vi "测量文件.vi"() -> ()   [LabVIEW 2016]
panel:
  out "数值 8":dbl
  out "数值 7":dbl
  out "数值 6":dbl
  out "数值 5":dbl
  out "动态显示 2":dbl[](array[numeric])
  out "动态显示":dbl[](array[numeric])
  out "数值 4":dbl
  out "数值 3":dbl
  out "数值 2":dbl
  out "数值":dbl
  in  "conversion rate(Hz)":dbl
  in  "停止":bool
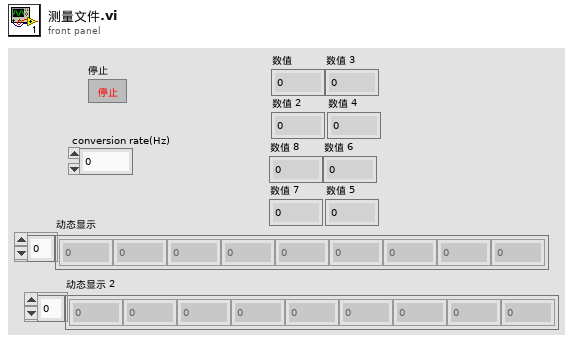
[diagram p1: front panel]
types:
  T1 = enum16{"open", "replace", "create", "open or create", "replace or create", "replace or create with confirmation"}
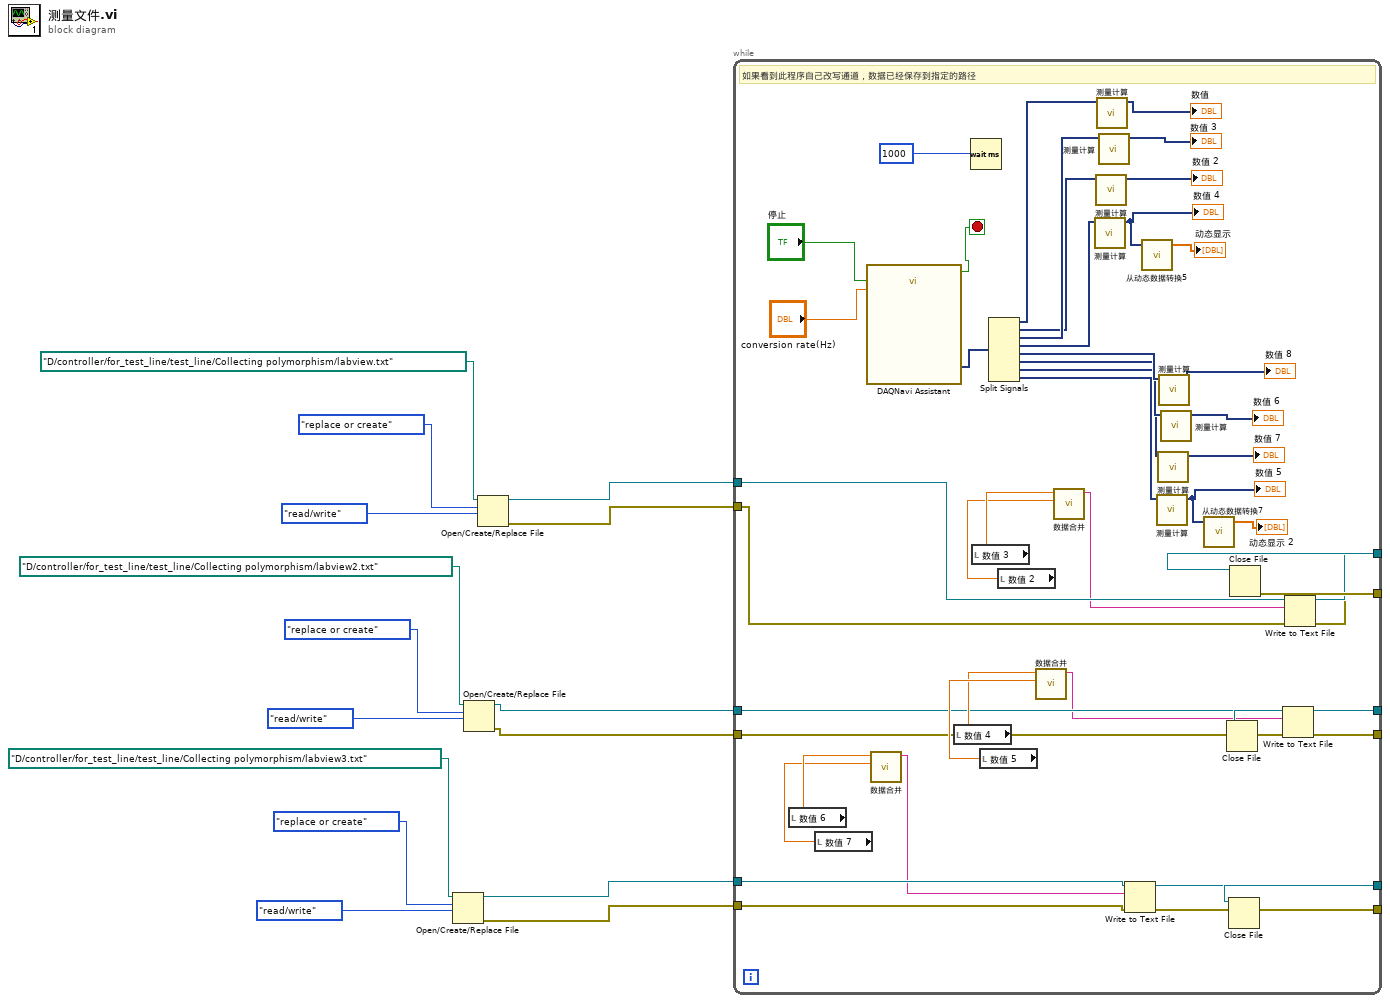
[diagram p0: block diagram]
diagram:
  n1 = Open/Create/Replace File(file path (use dialog)=path "D:/controller/for_test_line/test_line/Collecting polymorphism/labview3.txt" ("文件路径（使用对话框）"), operation (0:open)=T1."replace or create" ("操作(0:open)"), access (0:read/write)=enum16{"read/write", "read-only", "write-only"}."read/write" ("权限(0:read/write)")) -> (refnum out=w4:refnum<file>, error out=w3:errorcluster)  [unwired: 3 in, 1 out]
  n2 = Open/Create/Replace File(file path (use dialog)=path "D:/controller/for_test_line/test_line/Collecting polymorphism/labview2.txt" ("文件路径（使用对话框）"), operation (0:open)=T1."replace or create" ("操作(0:open)"), access (0:read/write)=enum16{"read/write", "read-only", "write-only"}."read/write" ("权限(0:read/write)")) -> (refnum out=w8:refnum<file>, error out=w7:errorcluster)  [unwired: 3 in, 1 out]
  n3 = Open/Create/Replace File(file path (use dialog)=path "D:/controller/for_test_line/test_line/Collecting polymorphism/labview.txt" ("文件路径（使用对话框）"), operation (0:open)=T1."replace or create" ("操作(0:open)"), access (0:read/write)=enum16{"read/write", "read-only", "write-only"}."read/write" ("权限(0:read/write)")) -> (refnum out=w21:refnum<file>, error out=w19:errorcluster)  [unwired: 3 in, 1 out]
  n4 = while {
    tunnel: w21 -> [w62]
    tunnel: [w61] -> w20
    tunnel: w19 -> [w60]
    tunnel: [w59] -> w18
    tunnel: w8 -> [w31]
    tunnel: w7 -> [w30]
    tunnel: [w29] -> w6
    tunnel: [w28] -> w5
    tunnel: w4 -> [w26]
    tunnel: w3 -> [w25]
    tunnel: [w24] -> w2
    tunnel: [w23] -> w1
    stop <- w63 stop-if-true
    # "如果看到此程序自己改写通道，数据已经保存到指定的路径"
    n5 = local read "数值 6"() -> (w33:dbl)
    n6 = local read "数值 7"() -> (w32:dbl)
    n7 = call "DAQNavi Assistant"("stop(true)"="停止", "conversion rate(Hz)"="conversion rate(Hz)") -> ("data out(DDT)"=w49:dynamicdata, "stopped"=w63:bool)  [unwired: 23 in, 1 out]
    n8 = call "数据合并.vi"("数值输入"=w32, "数值 3"=w33) -> ("字符串"=w22:string)  [unwired: 9 in]
    n9 = local read "数值 4"() -> (w34:dbl)
    n10 = Wait (ms)(milliseconds to wait=u32 1000 ("等待时间（毫秒）")) -> ()  [unwired: 1 out]
    n11 = local read "数值 3"() -> (w48:dbl)
    n12 = local read "数值 5"() -> (w35:dbl)
    n13 = Split Signals(w49) -> (w51:dynamicdata, w54:dynamicdata, w57:dynamicdata, w55:dynamicdata, w43:dynamicdata, w42:dynamicdata, w41:dynamicdata, w40:dynamicdata)  [unwired: 8 in]
    n14 = local read "数值 2"() -> (w45:dbl)
    n15 = call "数据合并.vi"("数值输入"=w35, "数值 3"=w34) -> ("字符串"=w27:string)  [unwired: 9 in]
    n16 = call "数据合并.vi"("数值输入"=w45, "数值 3"=w48) -> ("字符串"=w46:string)  [unwired: 9 in]
    n17 = call "测量计算.vi"("Dynamic Data输入"=w55) -> ("Dynamic Data输出"=w50:dynamicdata)  [unwired: 10 in]
    "数值 4" <- w50
    n18 = call "测量计算.vi"("Dynamic Data输入"=w54) -> ("Dynamic Data输出"=→"数值 2":dynamicdata)  [unwired: 10 in]
    n19 = call "测量计算.vi"("Dynamic Data输入"=w51) -> ("Dynamic Data输出"=→"数值":dynamicdata)  [unwired: 10 in]
    n20 = call "测量计算.vi"("Dynamic Data输入"=w57) -> ("Dynamic Data输出"=→"数值 3":dynamicdata)  [unwired: 10 in]
    n21 = Write to Text File(file (use dialog)=w26, text=w22, error in=w25) -> (refnum out=w24:refnum<file>, error out=w23:errorcluster)  [unwired: 1 in, 1 out]
    n22 = call "从动态数据转换5"("Dynamic Data Type"=w50) -> ("Array"=→"动态显示":dbl[])  [unwired: 3 in]
    n23 = call "测量计算.vi"("Dynamic Data输入"=w40) -> ("Dynamic Data输出"=w36:dynamicdata)  [unwired: 10 in]
    "数值 5" <- w36
    n24 = call "测量计算.vi"("Dynamic Data输入"=w41) -> ("Dynamic Data输出"=→"数值 7":dynamicdata)  [unwired: 10 in]
    n25 = call "测量计算.vi"("Dynamic Data输入"=w43) -> ("Dynamic Data输出"=→"数值 8":dynamicdata)  [unwired: 10 in]
    n26 = call "测量计算.vi"("Dynamic Data输入"=w42) -> ("Dynamic Data输出"=→"数值 6":dynamicdata)  [unwired: 10 in]
    n27 = call "从动态数据转换7"("Dynamic Data Type"=w36) -> ("Array"=→"动态显示 2":dbl[])  [unwired: 3 in]
    n28 = Write to Text File(file (use dialog)=w31, text=w27, error in=w30) -> (refnum out=w29:refnum<file>, error out=w28:errorcluster)  [unwired: 1 in, 1 out]
    n29 = Write to Text File(file (use dialog)=w62, text=w46, error in=w60) -> (refnum out=w61:refnum<file>, error out=w59:errorcluster)  [unwired: 1 in, 1 out]
  }
  n30 = Close File(refnum=w6, error in=w5) -> ()  [unwired: 2 out]
  n31 = Close File(refnum=w2, error in=w1) -> ()  [unwired: 2 out]
  n32 = Close File(refnum=w20, error in=w18) -> ()  [unwired: 2 out]
